vi "Convert Vector 3D (SGL) To UV 2D (SGL).vi"(11 "Vector 3D":T2) -> (3 "Point 2D":T1 {"v" min=0 max=1 step=0.1; "u" min=0 max=1 step=0.1})   [LabVIEW 2022 SP3, in "3D.lvlib"]
uses:
  3D.lvlib
  Vector 3D.ctl
  Raster/UV.ctl
  Raster/Raster.lvlib
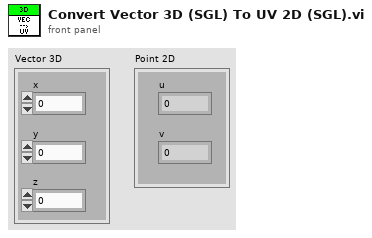
[diagram p1: front panel]
types:
  T1 = typedef "Raster.lvlib/UV.ctl" = cluster{"u":sgl, "v":sgl}
  T2 = typedef "3D.lvlib/Vector 3D.ctl" = cluster{"x":sgl, "y":sgl, "z":sgl}
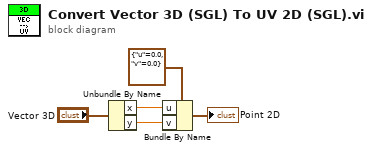
[diagram p0: block diagram]
diagram:
  n1 = Unbundle By Name("Vector 3D") -> ("x"=w2:sgl, "y"=w1:sgl)
  n2 = Bundle By Name(cluster=T1 {"u"=0.0, "v"=0.0} ("Point 2D"), "u"=w2, "v"=w1) -> (→"Point 2D":T1)
